vi "Move graph cursor.vi"(8 "error in (no error)":errorcluster, 9 "Coords":T2, 11 "Graph Ref in":T1) -> (0 "error out":errorcluster, 1 "Mouse coordinates":cluster{"X":dbl, "Y":dbl}, 2 "Graph cursor coordinates":cluster{"X":dbl, "Y":dbl}, 3 "Graph Ref out":T1)   [LabVIEW 2017, in "XGrapher.xctl"]
uses:
  XGrapher.xctl
  Typedefs/Xctrl-Timeline graph ref.ctl
  <vilib>/Utility/miscctls.llb/LVPoint32TypeDef.ctl
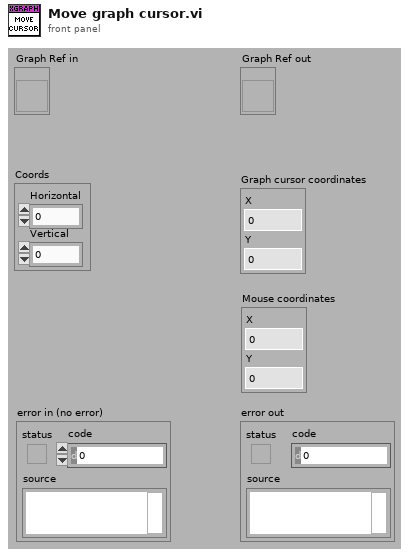
[diagram p1: front panel]
types:
  T1 = typedef "XGrapher.xctl/Xctrl-Timeline graph ref.ctl" = refnum<vi>
  T2 = typedef "LVPoint32TypeDef.ctl" = cluster{"Horizontal":i32, "Vertical":i32}
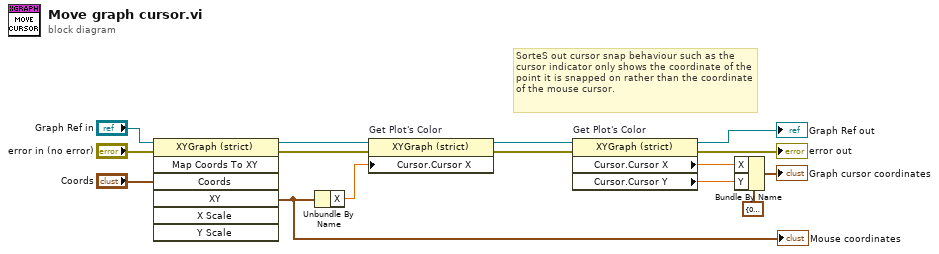
[diagram p0: block diagram]
diagram:
  # "SorteS out cursor snap behaviour such as the cursor indicator only shows the coordinate of the point it is snapped on rather than the coordinate of the mouse cursor."
  n1 = invoke on="Invoke Node" class="XYGraph (strict)" method="Map Coords To XY"(reference="Graph Ref in", error in="error in (no error)", "Coords"="Coords") -> (reference out=w11:T1, error out=w13:errorcluster, "XY"=w1:cluster{"X":dbl, "Y":dbl})  [unwired: 4 in, 4 out]
  "Mouse coordinates" <- w1
  n2 = Unbundle By Name(w1) -> ("X"=w2:dbl)
  n3 = property on="Get Plot's Color" class="XYGraph (strict)"(reference=w11, error in=w13, "Cursor.Cursor X"=w2) -> (reference out=w8:T1, error out=w4:errorcluster)
  n4 = property on="Get Plot's Color" class="XYGraph (strict)"(reference=w8, error in=w4) -> (reference out=→"Graph Ref out":T1, error out=→"error out":errorcluster, "Cursor.Cursor X"=w6:dbl, "Cursor.Cursor Y"=w5:dbl)
  n5 = Bundle By Name(cluster=cluster{"X":dbl, "Y":dbl} {"X"=0.0, "Y"=0.0} ("XY"), "X"=w6, "Y"=w5) -> (→"Graph cursor coordinates":cluster{"X":dbl, "Y":dbl})
